vi "ucno_numeric gradient.vi"(7 "function and data":T1, 8 "error in (no error)":errorcluster, 10 "f(X)":dbl=nan, 11 "X":dbl[](array[numeric])) -> (0 "error out":errorcluster, 2 "number of function evaluations":i32, 3 "gradient":dbl[](array[numeric]))   [LabVIEW 2017, in "NI_Gmath.lvlib"]
uses:
  NI_Gmath.lvlib
  ucno_user function ref and data.ctl
  ucno_user objective function ref.ctl
  fpuIEEE64_finiteDiffConstants.ctl
panel:
  in  "order":i32(ring)=1 items=["ORDER 1"=1, "ORDER 2"=2, "ORDER 4"=4]
  in  "stepsize (h)":dbl
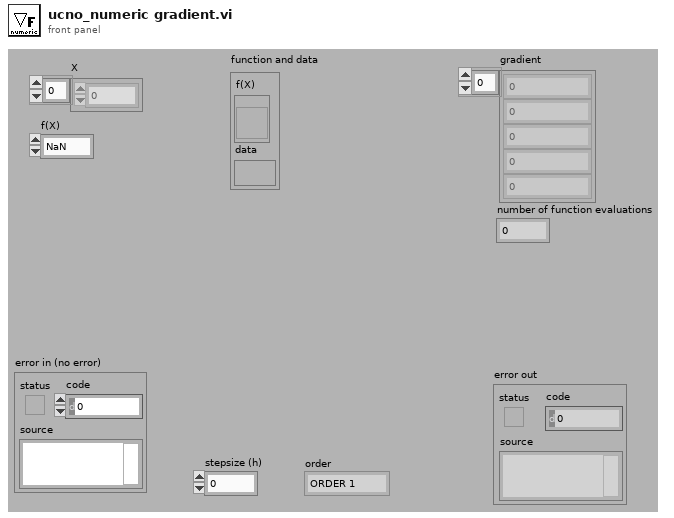
[diagram p1: front panel]
types:
  T1 = typedef "NI_Gmath.lvlib/ucno_user function ref and data.ctl" = cluster{"f(X)":T2, "data":variant}
  T2 = typedef "NI_Gmath.lvlib/ucno_user objective function ref.ctl" = refnum<vi>
  T3 = cluster{"objective function":bool, "gradient":bool}
  T4 = typedef "NI_Gmath.lvlib/fpuIEEE64_finiteDiffConstants.ctl" = dbl
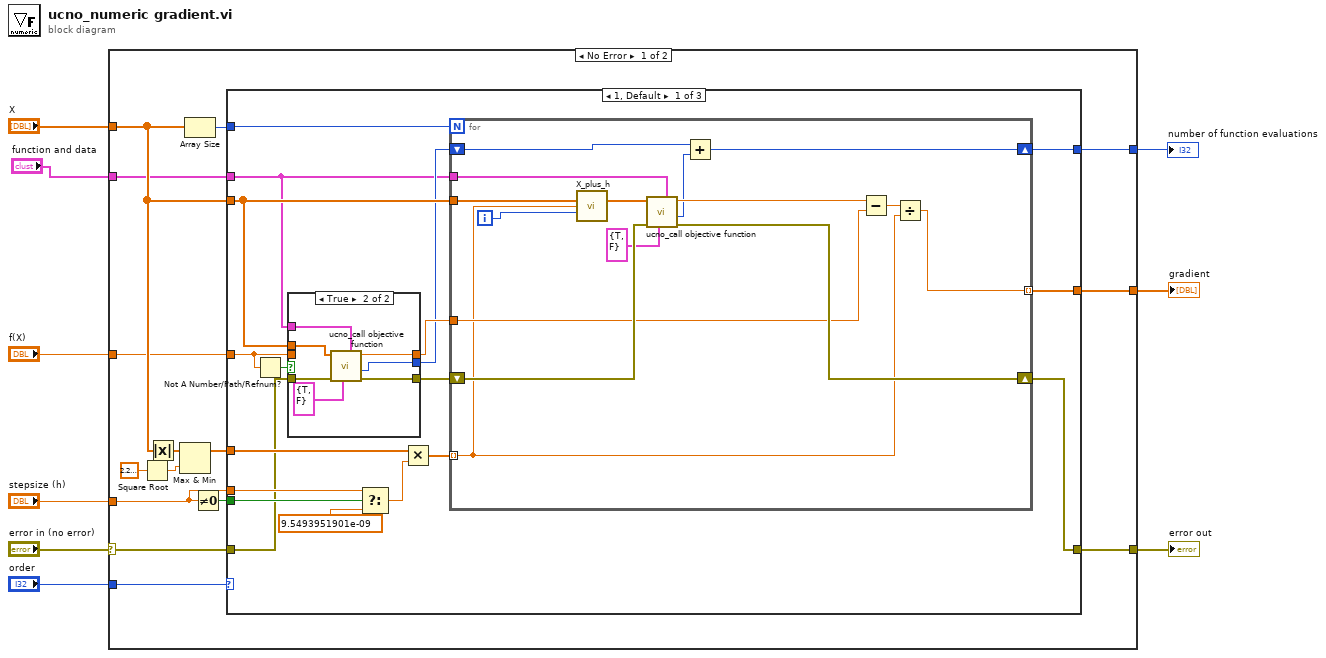
[diagram p0: block diagram]
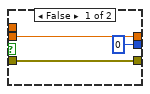
[diagram p2: hidden frame]
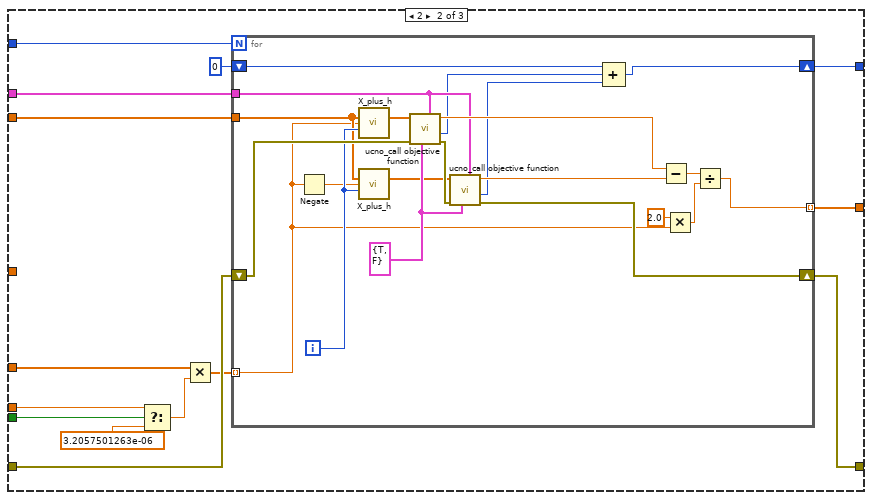
[diagram p3: hidden frame]
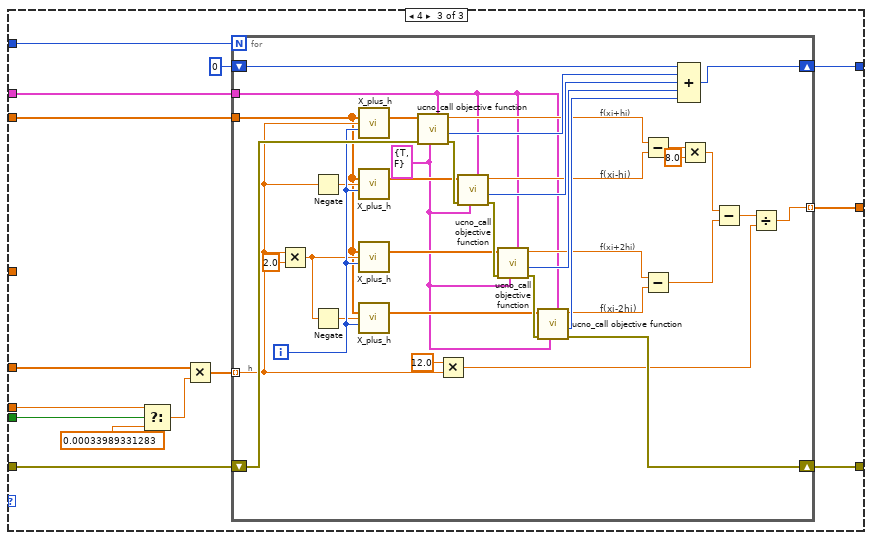
[diagram p4: hidden frame]
diagram:
  n1 = case shown="No Error" "error in (no error)" {
    selector: "error in (no error)" -> [w14 w153]
    tunnel: "X" -> [w24 _]
    tunnel: [w23 _] -> w8
    tunnel: "order" -> [w22 _]
    tunnel: "f(X)" -> [w20 _]
    tunnel: "stepsize (h)" -> [w19 _]
    tunnel: [w15 w153] -> w4
    tunnel: [w13 _] -> w2
    tunnel: "function and data" -> [w12 _]
    frame No Error {
      n2 = Square Root(x=2.220446049250313e-16) -> (sqrt(x)=w11:dbl)
      n3 = Absolute Value(x=w24) -> (abs(x)=w17:dbl[])
      n4 = Max & Min(x=w17, y=w11) -> (max(x,y)=w16:dbl[])  [unwired: 1 out]
      n5 = Array Size(array=w24) -> (size(s)=w21:i32)
      n6 = Not Equal To 0?(x=w19) -> (x != 0?=w18:bool)
      n7 = case shown="1, Default" w22 {
        tunnel: w24 -> [w38 w80 w116]
        tunnel: w14 -> [w28 w81 w107]
        tunnel: [w41 w79 w115] -> w23
        tunnel: w21 -> [w40 w78 w114]
        tunnel: w20 -> [w37 _ _]
        tunnel: w19 -> [w36 w75 w112]
        tunnel: w18 -> [w35 w76 w111]
        tunnel: w16 -> [w32 w74 w109]
        tunnel: [w42 w71 w106] -> w15
        tunnel: [w27 w69 w105] -> w13
        tunnel: w12 -> [w25 w68 w103]
        frame 1, Default {
          w34 = T4 9.5493951901e-09 items=["H_FINITE_DIFF_1"=9.5493951901e-09, "H_FINITE_DIFF_2"=3.2057501263e-06, "H_FINITE_DIFF_4"=0.00033989331283, "H_FINITE_DIFF_K_1"=2.8120287999e-06, "H_FINITE_DIFF_K_2"=9.1341513557e-05, "H_FINITE_DIFF_K_3"=0.00045180790895, "H_FINITE_DIFF_K_4"=0.0014917421406] ("fpuIEEE64")
          n8 = Not A Number/Path/Refnum?(number/path/refnum=w37) -> (NaN/Path/Refnum?=w30:bool)
          n9 = case shown="True" w30 {
            tunnel: [w45 w49] -> w39
            tunnel: w38 -> [_ w50]
            tunnel: w37 -> [w45 _]
            tunnel: w28 -> [w44 w52]
            tunnel: [w44 w51] -> w29
            tunnel: [0 ("number of function evaluations") w47] -> w26
            tunnel: w25 -> [_ w48]
            frame False {
            }
            frame True {
              n10 = call "ucno_call objective function.vi"("function and data"=w48, "output control"=T3 {"objective function"=TRUE, "gradient"=FALSE}, "error in (no error)"=w52, "X"=w50) -> ("error out"=w51:errorcluster, "number of function evaluations"=w47:i32, "f(X)"=w49:dbl)  [unwired: 4 in, 1 out]
            }
          }
          n11 = Select(t=w36, s=w35, f=w34) -> (s? t:f=w33:T4)
          n12 = Multiply(x=w32, y=w33) -> (x*y=w31:T4[])
          n13 = for {
            N: w40 -> [_]
            tunnel: w38 -> [w61]
            tunnel: [w65] -> w41 mode=indexing
            tunnel: w39 -> [w63]
            tunnel: w31 -> [w60] mode=indexing
            shift-right: [w66] -> w42
            shift-left: w29 -> [w67]
            shift-right: [w56] -> w27
            shift-left: w26 -> [w57]
            tunnel: w25 -> [w55]
            i -> [w62]
            n14 = call "X_plus_h.vi"("X"=w61, "h"=w60, "i"=w62) -> ("Xi+h"=w59:dbl[])  [unwired: 12 in]
            n15 = call "ucno_call objective function.vi"("function and data"=w55, "output control"=T3 {"objective function"=TRUE, "gradient"=FALSE}, "error in (no error)"=w67, "X"=w59) -> ("error out"=w66:errorcluster, "number of function evaluations"=w54:i32, "f(X)"=w58:dbl)  [unwired: 4 in, 1 out]
            n16 = Add(x=w57, y=w54) -> (x+y=w56:i32)
            n17 = Subtract(x=w58, y=w63) -> (x-y=w64:dbl)
            n18 = Divide(x=w64, y=w60) -> (x/y=w65:T4)
          }
        }
        frame 2 {
          w77 = T4 3.2057501263e-06 items=["H_FINITE_DIFF_1"=9.5493951901e-09, "H_FINITE_DIFF_2"=3.2057501263e-06, "H_FINITE_DIFF_4"=0.00033989331283, "H_FINITE_DIFF_K_1"=2.8120287999e-06, "H_FINITE_DIFF_K_2"=9.1341513557e-05, "H_FINITE_DIFF_K_3"=0.00045180790895, "H_FINITE_DIFF_K_4"=0.0014917421406] ("fpuIEEE64")
          n19 = Select(t=w75, s=w76, f=w77) -> (s? t:f=w73:T4)
          n20 = Multiply(x=w74, y=w73) -> (x*y=w72:T4[])
          n21 = for {
            N: w78 -> [_]
            tunnel: w80 -> [w93]
            tunnel: [w95] -> w79 mode=indexing
            tunnel: w72 -> [w92] mode=indexing
            shift-right: [w100] -> w71
            shift-left: w81 -> [w99]
            shift-right: [w85] -> w69
            shift-left: 0 -> [w86]
            tunnel: w68 -> [w84]
            i -> [w98]
            w102 = T3 {"objective function"=TRUE, "gradient"=FALSE} ("output control")
            n22 = Negate(x=w92) -> (-x=w91:T4)
            n23 = call "X_plus_h.vi"("X"=w93, "h"=w92, "i"=w98) -> ("Xi+h"=w90:dbl[])  [unwired: 12 in]
            n24 = call "X_plus_h.vi"("X"=w93, "h"=w91, "i"=w98) -> ("Xi+h"=w88:dbl[])  [unwired: 12 in]
            n25 = call "ucno_call objective function.vi"("function and data"=w84, "output control"=w102, "error in (no error)"=w99, "X"=w90) -> ("error out"=w101:errorcluster, "number of function evaluations"=w83:i32, "f(X)"=w89:dbl)  [unwired: 4 in, 1 out]
            n26 = call "ucno_call objective function.vi"("function and data"=w84, "output control"=w102, "error in (no error)"=w101, "X"=w88) -> ("error out"=w100:errorcluster, "number of function evaluations"=w82:i32, "f(X)"=w87:dbl)  [unwired: 4 in, 1 out]
            n27 = Compound Arithmetic op=ADD(w86, w83, w82) -> (w85:i32)
            n28 = Subtract(x=w89, y=w87) -> (x-y=w94:dbl)
            n29 = Multiply(x=2.0, y=w92) -> (x*y=w96:T4)
            n30 = Divide(x=w94, y=w96) -> (x/y=w95:T4)
          }
        }
        frame 4 {
          w113 = T4 0.00033989331283 items=["H_FINITE_DIFF_1"=9.5493951901e-09, "H_FINITE_DIFF_2"=3.2057501263e-06, "H_FINITE_DIFF_4"=0.00033989331283, "H_FINITE_DIFF_K_1"=2.8120287999e-06, "H_FINITE_DIFF_K_2"=9.1341513557e-05, "H_FINITE_DIFF_K_3"=0.00045180790895, "H_FINITE_DIFF_K_4"=0.0014917421406] ("fpuIEEE64")
          n31 = Select(t=w112, s=w111, f=w113) -> (s? t:f=w110:T4)
          n32 = Multiply(x=w109, y=w110) -> (x*y=w108:T4[])
          n33 = for {
            N: w114 -> [_]
            tunnel: w116 -> [w129]
            tunnel: [w135] -> w115 mode=indexing
            tunnel: w108 -> [w132] mode=indexing
            shift-right: [w147] -> w106
            shift-left: w107 -> [w148]
            shift-right: [w119] -> w105
            shift-left: 0 -> [w120]
            tunnel: w103 -> [w118]
            i -> [w143]
            w117 = T3 {"objective function"=TRUE, "gradient"=FALSE} ("output control")
            # "h"
            # "f(xi-2hi)"
            # "f(xi+2hi)"
            # "f(xi-hi)"
            # "f(xi+hi)"
            n34 = Multiply(x=w132, y=2.0) -> (x*y=w130:T4)
            n35 = Negate(x=w132) -> (-x=w134:T4)
            n36 = Negate(x=w130) -> (-x=w131:T4)
            n37 = call "X_plus_h.vi"("X"=w129, "h"=w132, "i"=w143) -> ("Xi+h"=w128:dbl[])  [unwired: 12 in]
            n38 = call "X_plus_h.vi"("X"=w129, "h"=w134, "i"=w143) -> ("Xi+h"=w125:dbl[])  [unwired: 12 in]
            n39 = call "X_plus_h.vi"("X"=w129, "h"=w130, "i"=w143) -> ("Xi+h"=w123:dbl[])  [unwired: 12 in]
            n40 = call "X_plus_h.vi"("X"=w129, "h"=w131, "i"=w143) -> ("Xi+h"=w121:dbl[])  [unwired: 12 in]
            n41 = call "ucno_call objective function.vi"("function and data"=w118, "output control"=w117, "error in (no error)"=w148, "X"=w128) -> ("error out"=w144:errorcluster, "number of function evaluations"=w149:i32, "f(X)"=w127:dbl)  [unwired: 4 in, 1 out]
            n42 = Multiply(x=12.0, y=w132) -> (x*y=w137:T4)
            n43 = call "ucno_call objective function.vi"("function and data"=w118, "output control"=w117, "error in (no error)"=w144, "X"=w125) -> ("error out"=w145:errorcluster, "number of function evaluations"=w150:i32, "f(X)"=w126:dbl)  [unwired: 4 in, 1 out]
            n44 = call "ucno_call objective function.vi"("function and data"=w118, "output control"=w117, "error in (no error)"=w145, "X"=w123) -> ("error out"=w146:errorcluster, "number of function evaluations"=w151:i32, "f(X)"=w124:dbl)  [unwired: 4 in, 1 out]
            n45 = call "ucno_call objective function.vi"("function and data"=w118, "output control"=w117, "error in (no error)"=w146, "X"=w121) -> ("error out"=w147:errorcluster, "number of function evaluations"=w152:i32, "f(X)"=w122:dbl)  [unwired: 4 in, 1 out]
            n46 = Subtract(x=w127, y=w126) -> (x-y=w141:dbl)
            n47 = Subtract(x=w124, y=w122) -> (x-y=w138:dbl)
            n48 = Compound Arithmetic op=ADD(w120, w149, w150, w151, w152) -> (w119:i32)
            n49 = Multiply(x=w141, y=8.0) -> (x*y=w139:dbl)
            n50 = Subtract(x=w139, y=w138) -> (x-y=w136:dbl)
            n51 = Divide(x=w136, y=w137) -> (x/y=w135:T4)
          }
        }
      }
    }
    frame Error {
    }
  }
  "error out" <- w4
  "gradient" <- w8
  "number of function evaluations" <- w2
